vi "Construct configuration database.vi"(8 "error in (no error)":errorcluster, 10 "SQL logic type":refnum<class "IConfigurationDatabaseQueries.lvclass">, 11 "Database type in":refnum<class "IDatabase.lvclass">) -> (0 "error out":errorcluster, 3 "database-configuration out":refnum<class "configuration-database.lvclass">)   [LabVIEW 2020, in "configuration-database.lvlib" / "configuration-database.lvclass"]
uses:
  configuration-database.lvclass
  externals/sqlite3/Source/sqlite3.lvclass
  sqlite-queries/sqlite-queries.lvclass
  externals/database-interface/IDatabase/IDatabase/IDatabase.lvclass
  IConfigDBQueries/IConfigurationDatabaseQueries.lvclass
  configuration-database.lvclass/configuration-database.ctl
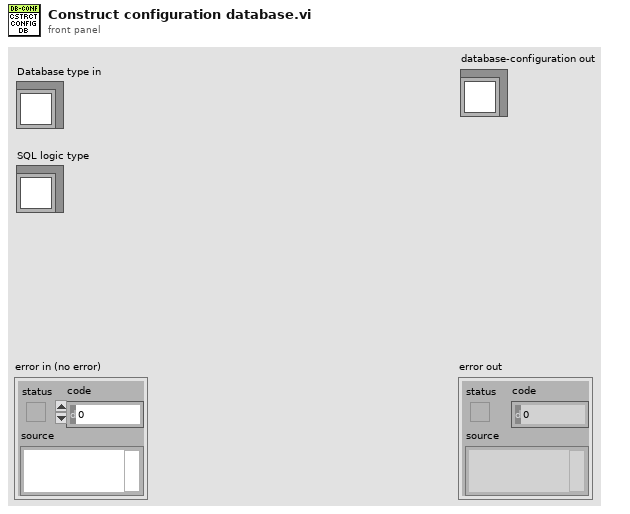
[diagram p1: front panel]
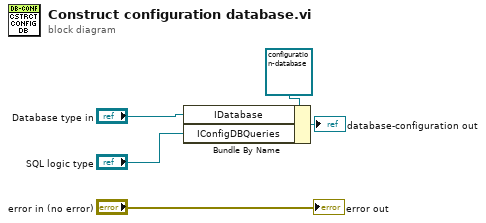
[diagram p0: block diagram]
diagram:
  n1 = Bundle By Name(cluster=refnum<class "configuration-database.lvclass"> refnum ("database-configuration in"), "IDatabase"="Database type in", "IConfigDBQueries"="SQL logic type") -> (→"database-configuration out":refnum<class "configuration-database.lvclass">)
  "error out" <- "error in (no error)"
